vi "enable_ddm_fets.vi"(6 "timeout (25000ms)":i32=25000, 8 "error in (no error)":errorcluster, 10 "On Period ms":u32, 11 "daemon reference in":refnum<k5>) -> (0 "error out":errorcluster, 2 "response":string, 3 "daemon reference out":refnum<k5>, 5 "command out":string="random")   [LabVIEW 2017]
doc: "<b>Command: </b>\"template\"\n\n<b>Description: </b> This command does something.\n\n<b>Parameters: </b> None\n____________________________________________\nDIPC 692 Daemon API 10.0.0.1\nSam Tee - Dyson Technology Ltd\nCopyright (c) 2024, Dyson Technology Ltd"
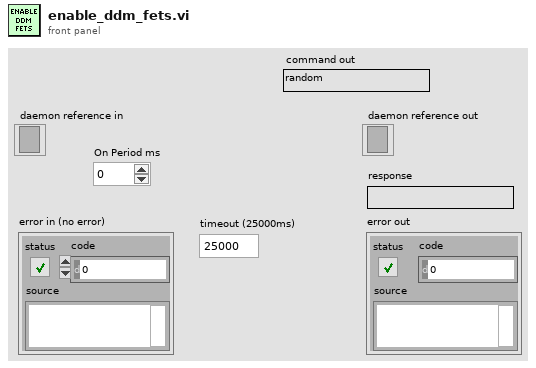
[diagram p1: front panel]
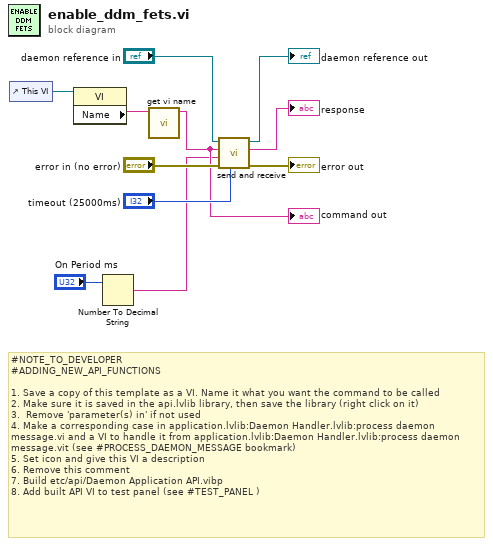
[diagram p0: block diagram]
diagram:
  # "#NOTE_TO_DEVELOPER\n#ADDING_NEW_API_FUNCTIONS\n\n1. Save a copy of this template as a VI. Name it what you want the command to be called\n2. Make sure it is saved in the api.lvlib library, then save the library (right click on it)\n3.  Remove 'parameter(s) in' if not used\n4. Make a corresponding case in application.lvlib:Daemon Handler.lvlib:process daemon message.vi and a VI to handle it from application.lvlib:Daemon Handler.lvlib:process daemon message.vit (see #PROCESS_DAEMON_MESSAGE bookmark)\n5. Set icon and give this VI a description\n6. Remove this comment\n7. Build etc/api/Daemon Application API.vibp\n8. Add built API VI to test panel (see #TEST_PANEL )"
  n1 = control-ref of="This VI"() -> (w5:refnum<vi>)
  n2 = property class="VI"(reference=w5) -> ("Name"=w4:string)  [unwired: 1 in, 2 out]
  n3 = Number To Decimal String(number="On Period ms") -> (decimal integer string=w1:string)  [unwired: 1 in]
  n4 = call "get vi name.vi"("library.lvlib:name.vi"=w4) -> ("vi name"=w3:string)  [unwired: 10 in]
  "command out" <- w3
  n5 = call "send and receive.vi"("timeout (25000ms)"="timeout (25000ms)", "error in (no error)"="error in (no error)", "data"=w1, "command"=w3, "daemon reference in"="daemon reference in") -> ("error out"=→"error out":errorcluster, "response"=→"response":string, "daemon reference out"=→"daemon reference out":refnum<k5>)  [unwired: 4 in]
